vi "PRM1Z8_Init.vi"(8 "error in (no error)":errorcluster) -> (0 "error out":errorcluster, 3 "reference out":refnum<k24>)   [LabVIEW 2018, in "Laser Quantum.lvlib"]
uses:
  Laser Quantum.lvlib
  C:/Program Files/Thorlabs/Kinesis/ThorLabs.MotionControl.KCube.DCServoCLI.dll
  Program Files/Thorlabs/Kinesis/ThorLabs.MotionControl.KCube.DCServoCLI.dll
  C:/Program Files/Thorlabs/Kinesis/Thorlabs.MotionControl.DeviceManagerCLI.dll
  Program Files/Thorlabs/Kinesis/Thorlabs.MotionControl.DeviceManagerCLI.dll
  C:/Program Files/Thorlabs/Kinesis/Thorlabs.MotionControl.GenericMotorCLI.dll
  Program Files/Thorlabs/Kinesis/Thorlabs.MotionControl.GenericMotorCLI.dll
panel:
  out "Controller Information":T1
  out "Device list (serial no.)":string[](array[string])
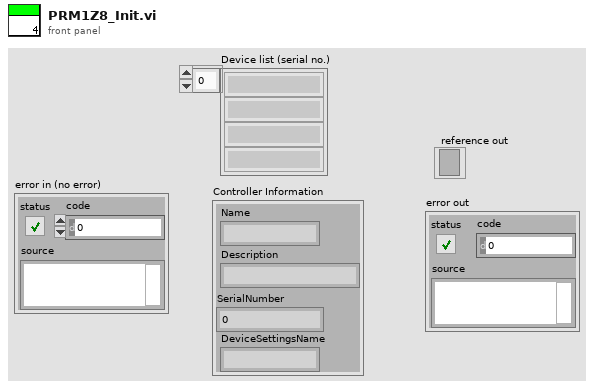
[diagram p1: front panel]
types:
  T1 = cluster{"Name":string, "Description":string, "SerialNumber":u32, "DeviceSettingsName":string}
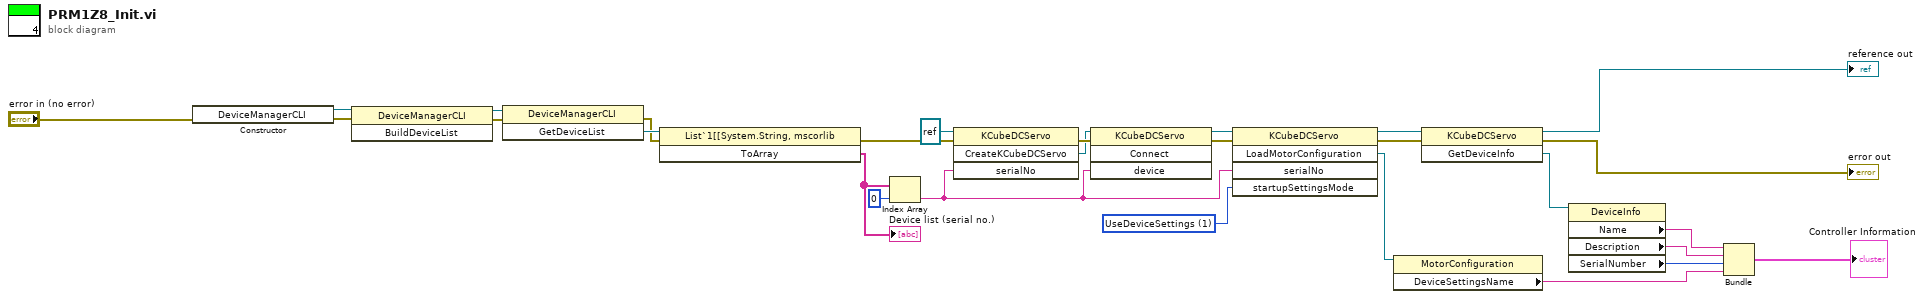
[diagram p0: block diagram]
diagram:
  w21 = 1 items=["UseDeviceSettings"=1, "UseFileSettings"=2, "UseConfiguredSettings"=3] ("startupSettingsMode")
  n1 = constructor class="DeviceManagerCLI"(error in="error in (no error)") -> (reference out=w18:refnum<k24>, error out=w1:errorcluster)  [unwired: 2 in, 1 out]
  n2 = invoke class="DeviceManagerCLI" method="BuildDeviceList"(reference=w18, error in=w1) -> (reference out=w15:refnum<k24>, error out=w17:errorcluster)  [unwired: 1 in, 1 out]
  n3 = invoke class="DeviceManagerCLI" method="GetDeviceList"(reference=w15, error in=w17) -> (error out=w14:errorcluster, "GetDeviceList"=w16:refnum<k24>)  [unwired: 1 in, 1 out]
  n4 = invoke class="List`1[[System.String, mscorlib" method="ToArray"(reference=w16, error in=w14) -> (error out=w13:errorcluster, "ToArray"=w12:string[])  [unwired: 1 in, 1 out]
  "Device list (serial no.)" <- w12
  n5 = Index Array(array=w12, index=0) -> (element=w10:string)
  n6 = invoke class="KCubeDCServo" method="CreateKCubeDCServo"(reference=refnum<k24> refnum ("target class"), error in=w13, "serialNo"=w10) -> (error out=w23:errorcluster, "CreateKCubeDCServo"=w22:refnum<k24>)  [unwired: 1 in, 2 out]
  n7 = invoke class="KCubeDCServo" method="Connect"(reference=w22, error in=w23, "device"=w10) -> (reference out=w20:refnum<k24>, error out=w19:errorcluster)  [unwired: 1 in, 2 out]
  n8 = invoke class="KCubeDCServo" method="LoadMotorConfiguration"(reference=w20, error in=w19, "serialNo"=w10, "startupSettingsMode"=w21) -> (reference out=w4:refnum<k24>, error out=w3:errorcluster, "LoadMotorConfiguration"=w2:refnum<k24>)  [unwired: 1 in, 2 out]
  n9 = property class="MotorConfiguration"(reference=w2) -> ("DeviceSettingsName"=w9:string)  [unwired: 1 in, 2 out]
  n10 = invoke class="KCubeDCServo" method="GetDeviceInfo"(reference=w4, error in=w3) -> (reference out=→"reference out":refnum<k24>, error out=→"error out":errorcluster, "GetDeviceInfo"=w5:refnum<k24>)  [unwired: 1 in]
  n11 = property class="DeviceInfo"(reference=w5) -> ("Name"=w6:string, "Description"=w7:string, "SerialNumber"=w8:u32)  [unwired: 1 in, 2 out]
  n12 = Bundle("Name"=w6, "Description"=w7, "SerialNumber"=w8, "DeviceSettingsName"=w9) -> (→"Controller Information":T1)  [unwired: 1 in]
